vi "m1m3_logEvent_ForceSetpointWarning.vi"(8 "error in (no error)":errorcluster, 11 "logevent_ForceSetpointWarning_Ctl":T1) -> (0 "error out":errorcluster, 2 "function return":i32, 3 "logevent_ForceSetpointWarning_Ctl out":T1)   [LabVIEW 2016, in "SALLV_m1m3.lvlib"]
doc: "int m1m3_shm_logEvent_ForceSetpointWarningLV(m1m3_logevent_ForceSetpointWarningLV *logevent_ForceSetpointWarning_Ctl );"
uses:
  SALLV_m1m3.lvlib
  DataTypes/logevent_ForceSetpointWarning.ctl
  SALLV_m1m3.so
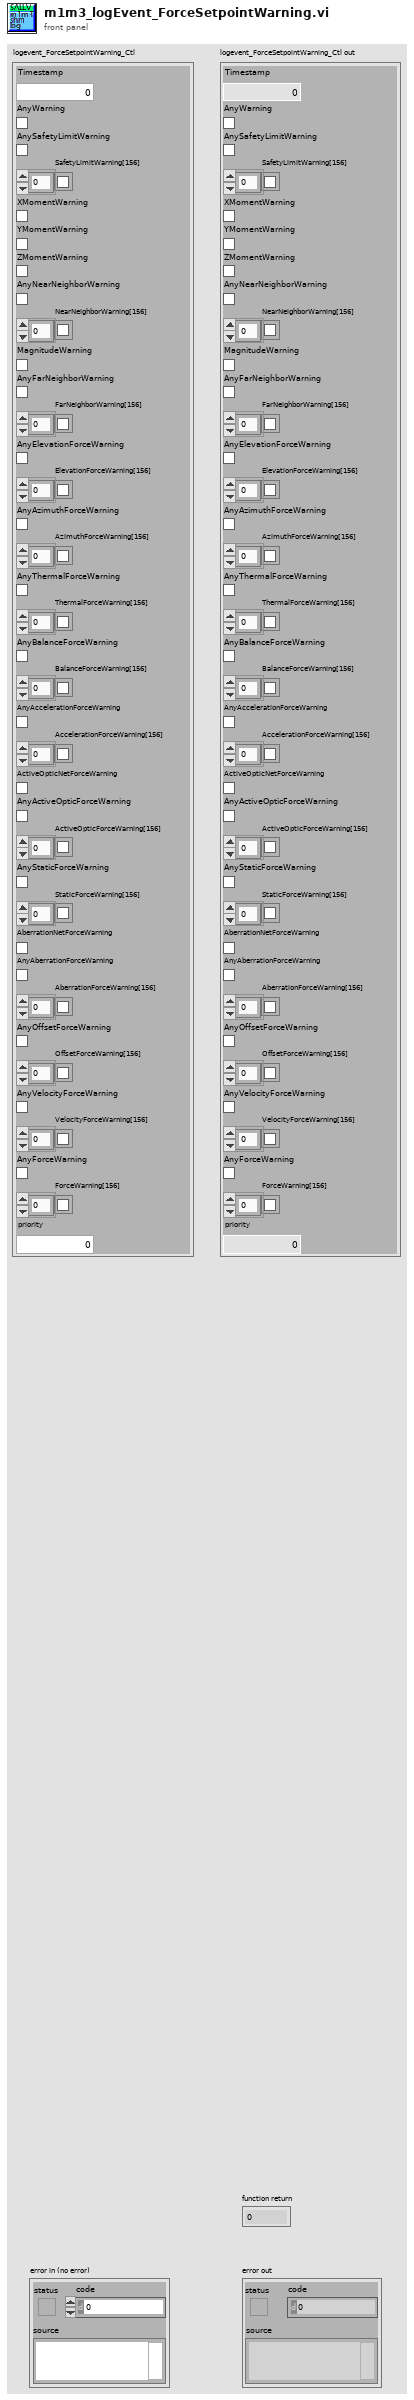
[diagram p1: front panel]
types:
  T1 = typedef "SALLV_m1m3.lvlib/logevent_ForceSetpointWarning.ctl" = cluster{"Timestamp":dbl, "AnyWarning":bool, "AnySafetyLimitWarning":bool, "SafetyLimitWarning[156]":bool[], "XMomentWarning":bool, "YMomentWarning":bool, "ZMomentWarning":bool, "AnyNearNeighborWarning":bool, "NearNeighborWarning[156]":bool[], "MagnitudeWarning":bool, "AnyFarNeighborWarning":bool, "FarNeighborWarning[156]":bool[], "AnyElevationForceWarning":bool, "ElevationForceWarning[156]":bool[], "AnyAzimuthForceWarning":bool, "AzimuthForceWarning[156]":bool[], "AnyThermalForceWarning":bool, "ThermalForceWarning[156]":bool[], "AnyBalanceForceWarning":bool, "BalanceForceWarning[156]":bool[], "AnyAccelerationForceWarning":bool, "AccelerationForceWarning[156]":bool[], "ActiveOpticNetForceWarning":bool, "AnyActiveOpticForceWarning":bool, "ActiveOpticForceWarning[156]":bool[], "AnyStaticForceWarning":bool, "StaticForceWarning[156]":bool[], "AberrationNetForceWarning":bool, "AnyAberrationForceWarning":bool, "AberrationForceWarning[156]":bool[], "AnyOffsetForceWarning":bool, "OffsetForceWarning[156]":bool[], "AnyVelocityForceWarning":bool, "VelocityForceWarning[156]":bool[], "AnyForceWarning":bool, "ForceWarning[156]":bool[], "priority":i32}
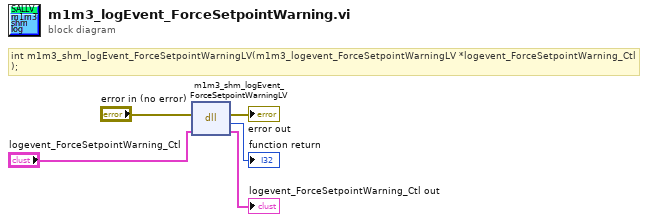
[diagram p0: block diagram]
diagram:
  # "int m1m3_shm_logEvent_ForceSetpointWarningLV(m1m3_logevent_ForceSetpointWarningLV *logevent_ForceSetpointWarning_Ctl );"
  n1 = dll-call lib="opt/CODE/SALLV_m1m3/SALLV_m1m3.*" fn="m1m3_shm_logEvent_ForceSetpointWarningLV"(error in="error in (no error)", "logevent_ForceSetpointWarning_Ctl"="logevent_ForceSetpointWarning_Ctl") -> (error out=→"error out":errorcluster, →"function return":i32, "logevent_ForceSetpointWarning_Ctl"=→"logevent_ForceSetpointWarning_Ctl out":T1)  [unwired: 2 in, 1 out]
